vi "Configure Active Trace.vi"(8 "error in (no error)":errorcluster, 10 "Active Trace Number (1)":u16=1 min=1, 11 "MXA in":refnum<class "MXA.lvclass">) -> (0 "error out":errorcluster, 3 "MXA out":refnum<class "MXA.lvclass">)   [LabVIEW 2020, in "MXA.lvclass"]
uses:
  MXA.lvclass
  C:/Sandbox/RF Bench/Source Code/WiSpry Test Framework/Instruments/Instrument.lvclass
  C:/Sandbox/RF Bench/Source Code/WiSpry Test Framework/Instruments/Spectrum Analyzer/Spectrum Analyzer.lvclass
  Instrument.lvclass/Instrument.ctl
  Spectrum Analyzer.lvclass/Spectrum Analyzer.ctl
  Instrument.lvclass
  <instrlib>/Agilent MXA Series/Agilent MXA Series.lvlib
  Spectrum Analyzer.lvclass
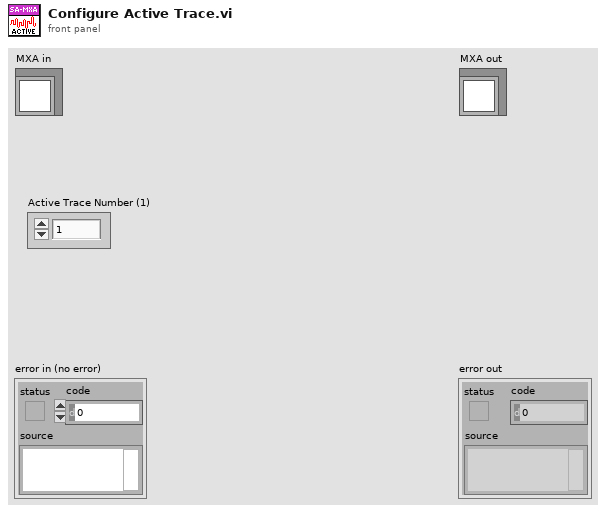
[diagram p1: front panel]
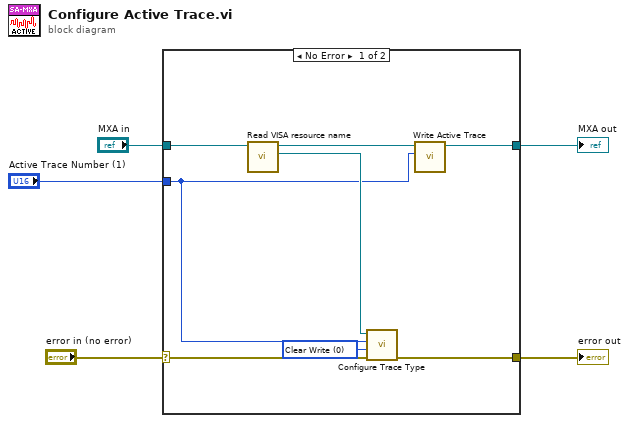
[diagram p0: block diagram]
diagram:
  n1 = case shown="No Error" "error in (no error)" {
    selector: "error in (no error)" -> [w10 w15]
    tunnel: "MXA in" -> [w13 w14]
    tunnel: [w9 w15] -> w4
    tunnel: [w7 w14] -> w3
    tunnel: "Active Trace Number (1)" -> [w6 _]
    frame No Error {
      w11 = 0 items=["Clear Write", "Average", "Maximum Hold", "Minimum Hold"] ("Trace Type (0: Clear Write)")
      n2 = call "Read VISA resource name.vi"("Instrument in"=w13) -> ("VISA resource name"=w12:refnum<visa-resource-name>, "Instrument out"=w8:refnum<class "MXA.lvclass">)  [unwired: 9 in]
      n3 = call <instrlib>:"Configure Trace Type.vi"("error in (no error)"=w10, "Trace Type (0: Clear Write)"=w11, "Trace Name (1: Trace 1)"=w6, "VISA resource name"=w12) -> ("error out"=w9:errorcluster)  [unwired: 6 in, 1 out]
      n4 = call "Write Active Trace.vi"("Active Trace"=w6, "Spectrum Analyzer in"=w8) -> ("Spectrum Analyzer out"=w7:refnum<class "MXA.lvclass">)  [unwired: 9 in]
    }
    frame Error {
    }
  }
  "error out" <- w4
  "MXA out" <- w3
